vi "WF3154 4Ch Fault Injection.vi"(2 "Packet (1)":u64, 4 "WF-3154 IO":T1={"WF-3154 CH0"="WF-3154/CH0", "WF-3154 CH1"="WF-3154/CH1", "WF-3154 CH2"="WF-3154/CH2", "WF-3154 CH3"="WF-3154/CH3"}) -> ()   [LabVIEW 2010]
doc: "This VI should be used together with the WF-3154 when creating a custom FPGA for VeriStand.\nIt uses one (1) packet."
uses:
  <vilib>/eio/EIONode/EIONode.xnode
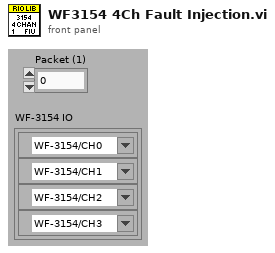
[diagram p1: front panel]
types:
  T1 = cluster{"WF-3154 CH0":refnum<k21>, "WF-3154 CH1":refnum<k21>, "WF-3154 CH2":refnum<k21>, "WF-3154 CH3":refnum<k21>}
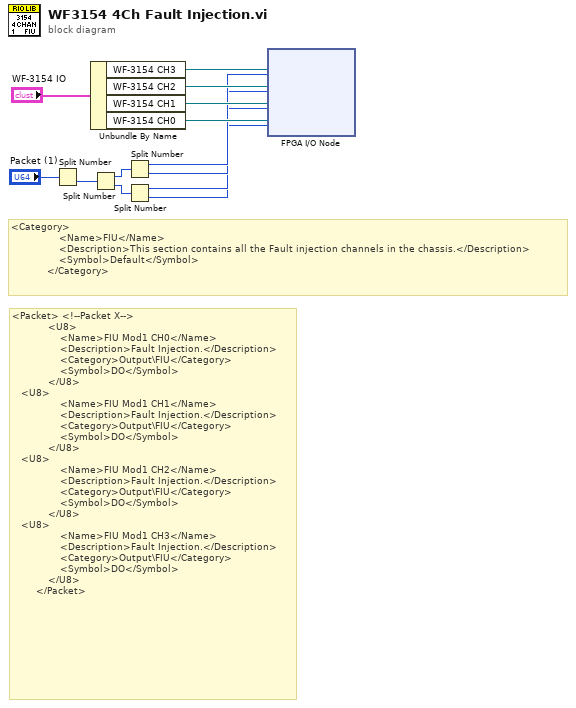
[diagram p0: block diagram]
diagram:
  # "<Packet>\t<!--Packet X-->\n            <U8>\n                <Name>FIU Mod1 CH0</Name>\n                <Description>Fault Injection.</Description>\n                <Category>Output\\FIU</Category>\n                <Symbol>DO</Symbol>\n            </U8>\n\t\t\t<U8>\n                <Name>FIU Mod1 CH1</Name>\n                <Description>Fault Injection.</Description>\n                <Category>Output\\FIU</Category>\n                <Symbol>DO</Symbol>\n            </U8>\n\t\t\t<U8>\n                <Name>FIU Mod1 CH2</Name>\n                <Description>Fault Injection.</Description>\n                <Category>Output\\FIU</Category>\n                <Symbol>DO</Symbol>\n            </U8>\n\t\t\t<U8>\n                <Name>FIU Mod1 CH3</Name>\n                <Description>Fault Injection.</Description>\n                <Category>Output\\FIU</Category>\n                <Symbol>DO</Symbol>\n            </U8>\n        </Packet>"
  # "<Category>\n                <Name>FIU</Name>\n                <Description>This section contains all the Fault injection channels in the chassis.</Description>\n                <Symbol>Default</Symbol>\n            </Category>"
  n1 = Split Number(x="Packet (1)") -> (lo(x)=w5:u32)  [unwired: 1 out]
  n2 = Unbundle By Name("WF-3154 IO") -> ("WF-3154 CH3"=w6:refnum<k21>, "WF-3154 CH2"=w7:refnum<k21>, "WF-3154 CH1"=w8:refnum<k21>, "WF-3154 CH0"=w9:refnum<k21>)
  n3 = Split Number(x=w5) -> (hi(x)=w12:u16, lo(x)=w13:u16)
  n4 = Split Number(x=w12) -> (hi(x)=w4:u8, lo(x)=w3:u8)
  n5 = Split Number(x=w13) -> (hi(x)=w2:u8, lo(x)=w1:u8)
  n6 = xnode "FPGA I/O Node"("I/O Item"=w4, "FPGA I/O In"=w6, "I/O Item"=w3, "FPGA I/O In"=w7, "I/O Item"=w2, "FPGA I/O In"=w8, "I/O Item"=w1, "FPGA I/O In"=w9) -> ()  [unwired: 4 out]
